vi "Get Features DB.vi"(6 "Local Data in":T3, 7 "UI References":T1, 8 "error in (no error)":errorcluster, 10 "Action":T2=enum."Get Preview", 11 "Mouse Position (Start)":cluster{"X":i32, "Y":i32}) -> (0 "error out":errorcluster, 1 "Refresh?":bool, 2 "Features":string[][](array[string]), 3 "FTR Names":string[](array[string]), 4 "Local Data out":T3)   [LabVIEW 2024]
uses:
  Controls/RVHR - Local Data.ctl
  Controls/Test Cluster.ctl
  Controls/Excluded Information.ctl
  Controls/Language.ctl
  Controls/Device_Type.ctl
  <vilib>/Utility/miscctls.llb/LVRectTypeDef.ctl
  <vilib>/Utility/miscctls.llb/LVBoundsTypeDef.ctl
  Controls/DB Manager Commands.ctl
  Controls/RVHR - UI Refs.ctl
  Controls/Run Listbox Command.ctl
  <vilib>/drjdpowell/SQLite Library/SQL Connection/Open (path).vi
  <vilib>/drjdpowell/SQLite Library/SQL Connection/Open (string).vi
  <vilib>/AdvancedString/Path To Command Line String.vi
  <vilib>/drjdpowell/SQLite Library/SQL Connection/Execute SQL (Single Integer).vi
  <vilib>/drjdpowell/SQLite Library/SQL Connection/Execute SQL.vi
  <vilib>/drjdpowell/SQLite Library/SQL Connection/Execute SQL (1D String).vi
  <vilib>/drjdpowell/SQLite Library/SQL Connection/Execute SQL (No results).vi
  <vilib>/drjdpowell/SQLite Library/SQL Connection/Connection.lvclass
  <vilib>/drjdpowell/SQLite Library/SQLite.lvlib
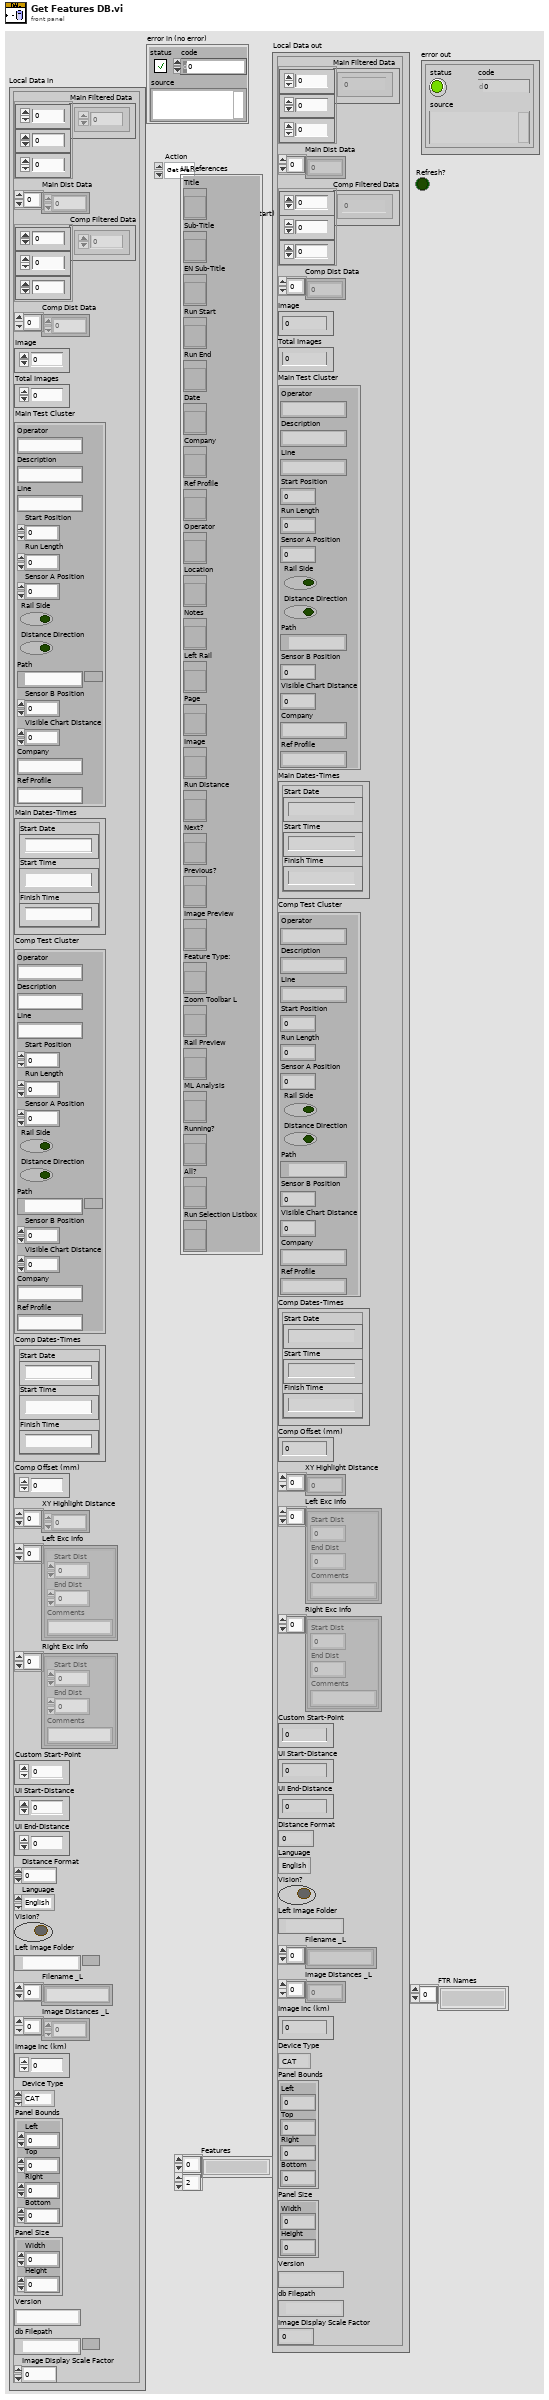
[diagram p1: front panel]
types:
  T1 = typedef "RVHR - UI Refs.ctl" = cluster{"Title":refnum<vi>, "Sub-Title":refnum<vi>, "EN Sub-Title":refnum<vi>, "Run Start":refnum<vi>, "Run End":refnum<vi>, "Date":refnum<vi>, "Company":refnum<vi>, "Ref Profile":refnum<vi>, "Operator":refnum<vi>, "Location":refnum<vi>, "Notes":refnum<vi>, "Left Rail":refnum<vi>, "Page":refnum<vi>, "Image":refnum<vi>, "Run Distance":refnum<vi>, "Next?":refnum<vi>, "Previous?":refnum<vi>, "Image Preview":refnum<vi>, "Feature Type:":refnum<vi>, "Zoom Toolbar L":refnum<vi>, "Rail Preview":refnum<vi>, "ML Analysis":refnum<vi>, "Running?":refnum<vi>, "All?":refnum<vi>, "Run Selection Listbox":refnum<vi>}
  T2 = typedef "DB Manager Commands.ctl" = enum16{"Get Image", "Get Preview", "Add", "Remove", "Update", "Get FTR Names"}
  T3 = typedef "RVHR - Local Data.ctl" = cluster{"Main Filtered Data":dbl[][][], "Main Dist Data":dbl[], "Comp Filtered Data":dbl[][][], "Comp Dist Data":dbl[], "Image":u16, "Total Images":u16, "Main Test Cluster":T4, "Main Dates-Times":cluster{"Start Date":string, "Start Time":string, "Finish Time":string}, "Comp Test Cluster":T4, "Comp Dates-Times":cluster{"Start Date":string, "Start Time":string, "Finish Time":string}, "Comp Offset (mm)":i64, "XY Highlight Distance":dbl[], "Left Exc Info":T5[], "Right Exc Info":T5[], "Custom Start-Point":dbl, "UI Start-Distance":dbl, "UI End-Distance":dbl, "Distance Format":u8, "Language":T6, "Vision?":bool, "Left Image Folder":path, "Filename _L":string[], "Image Distances _L":dbl[], "Image Inc (km)":dbl, "Device Type":T7, "Panel Bounds":T8, "Panel Size":T9, "Version":string, "db Filepath":path, "Image Display Scale Factor":dbl}
  T4 = typedef "Test Cluster.ctl" = cluster{"Operator":string, "Description":string, "Line":string, "Start Position":dbl, "Run Length":dbl, "Sensor A Position":dbl, "Rail Side":bool, "Distance Direction":bool, "Path":path, "Sensor B Position":dbl, "Visible Chart Distance":dbl, "Company":string, "Ref Profile":string}
  T5 = typedef "Excluded Information.ctl" = cluster{"Start Dist":dbl, "End Dist":dbl, "Comments":string}
  T6 = typedef "Language.ctl" = enum16{"English", "Chinese", "German"}
  T7 = typedef "Device_Type.ctl" = enum16{"CAT", "Bi-CAT", "YRCA", "RCA", "RV-HR", "TV-HR"}
  T8 = typedef "LVRectTypeDef.ctl" = cluster{"Left":i16, "Top":i16, "Right":i16, "Bottom":i16}
  T9 = typedef "LVBoundsTypeDef.ctl" = cluster{"Width":u32, "Height":u32}
  T10 = typedef "Run Listbox Command.ctl" = enum16{"Init", "Item Names", "Update", "Update All", "Get Selections", "Clear"}
  T11 = typedef "LVMouseTypeDef.ctl" = cluster{"Mouse Position":cluster{"X":i32, "Y":i32}, "Mouse Modifiers":cluster{"Button Down":bool, "Shift Mod":bool, "Menu Mod":bool, "Option Mod":bool}}
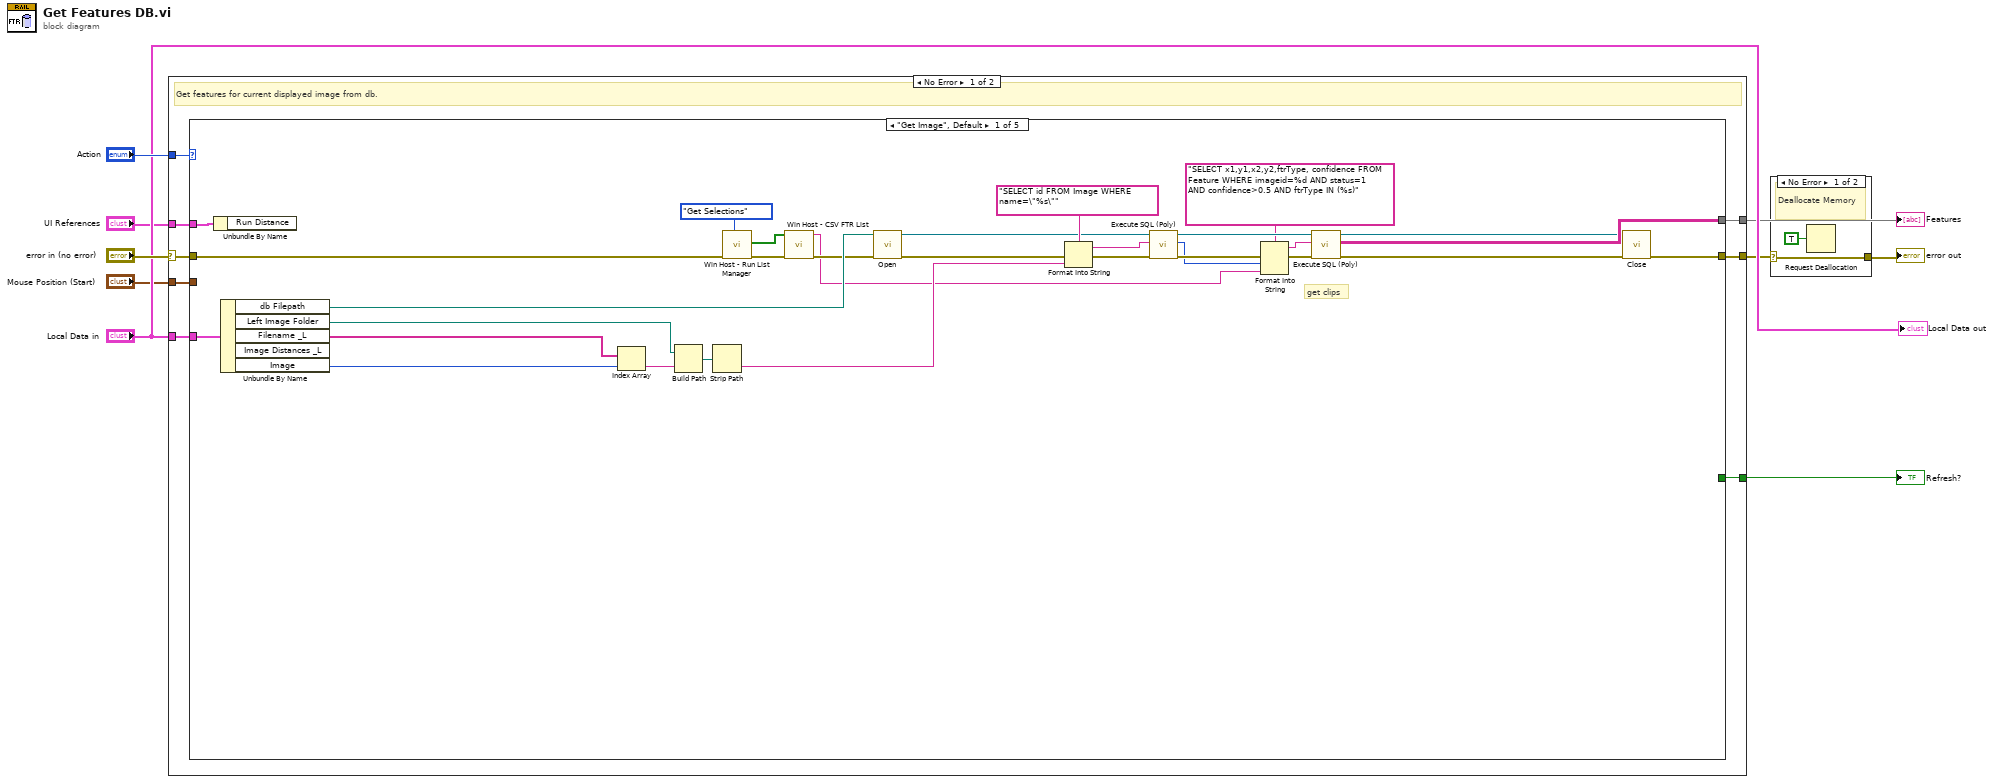
[diagram p0: block diagram]
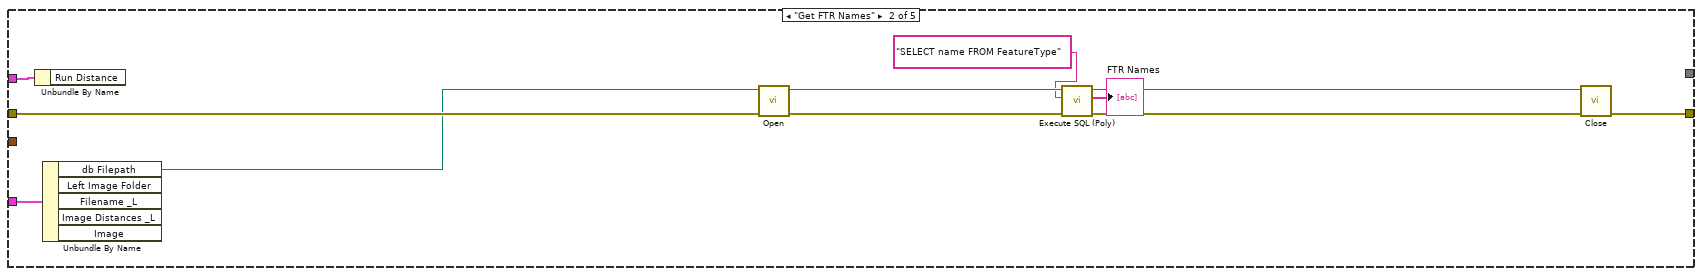
[diagram p3: hidden frame]
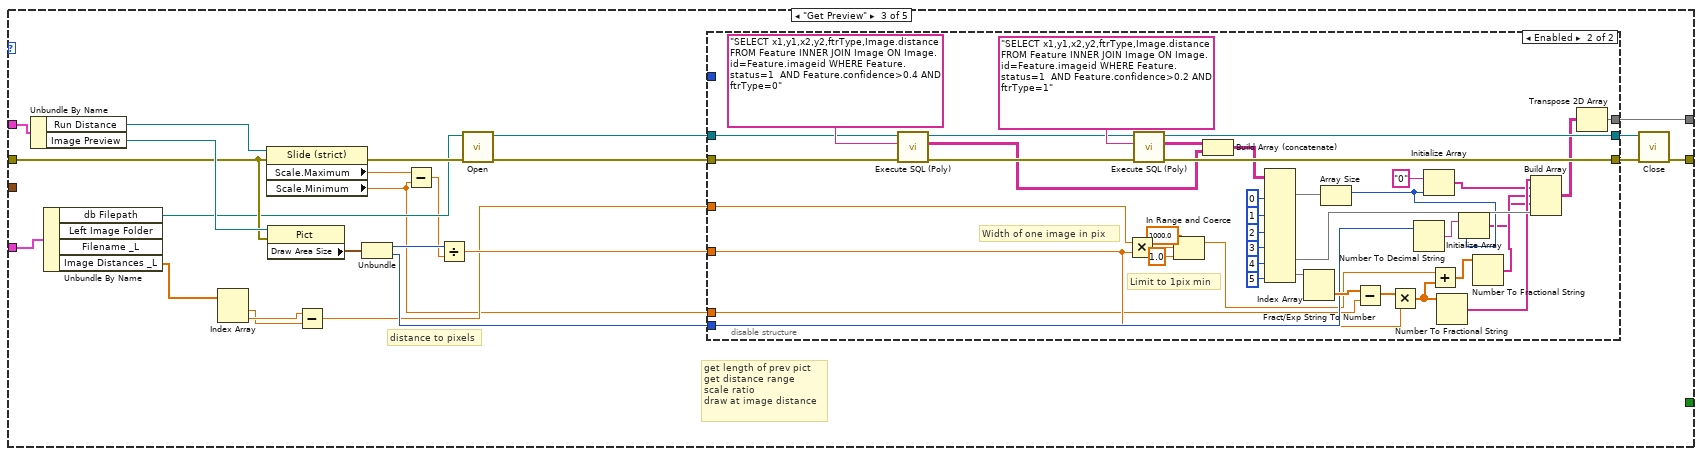
[diagram p4: hidden frame]
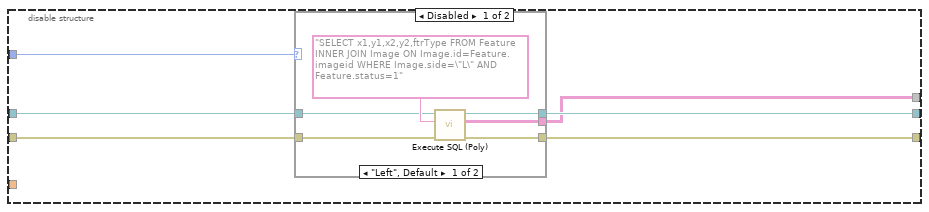
[diagram p5: hidden frame]
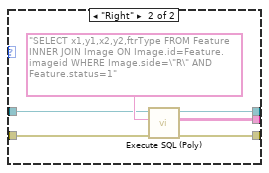
[diagram p6: hidden frame]
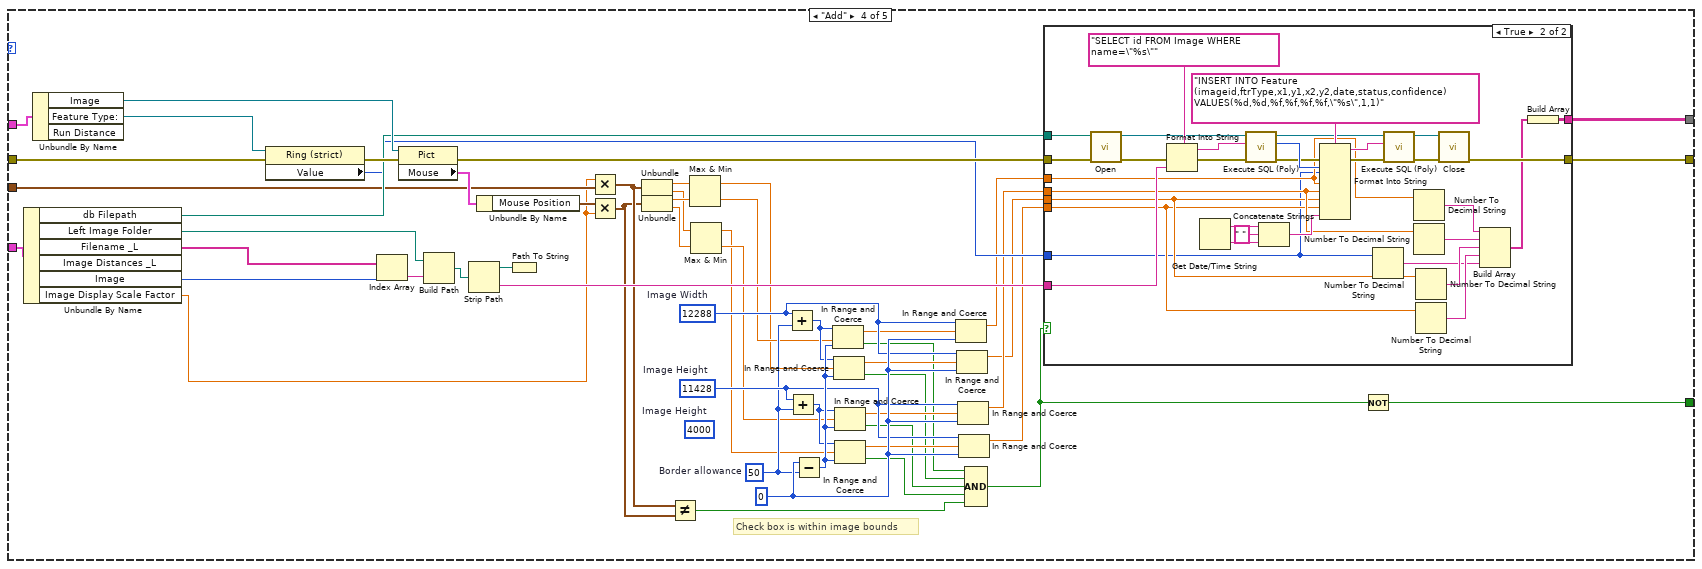
[diagram p7: hidden frame]
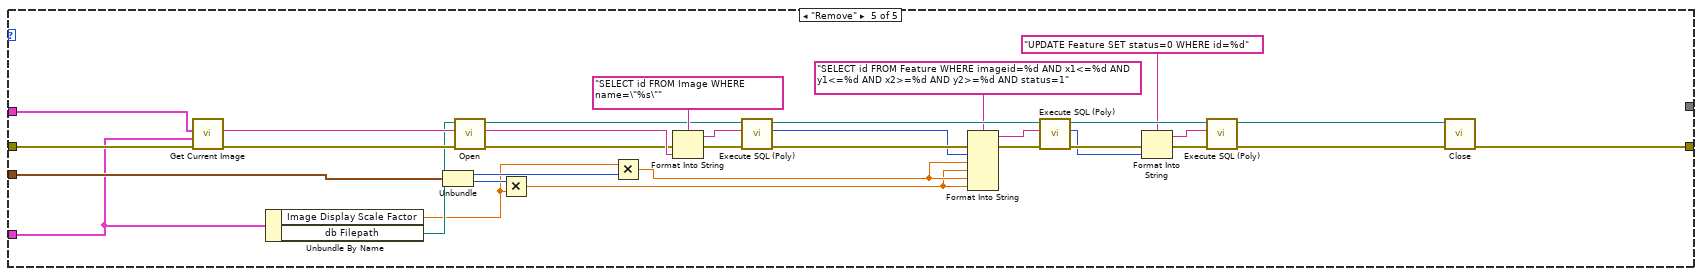
[diagram p9: hidden frame]
diagram:
  n1 = case shown="No Error" "error in (no error)" {
    selector: "error in (no error)" -> [w17 w262]
    tunnel: "Local Data in" -> [w15 _]
    tunnel: [w16 w262] -> w2
    tunnel: "Action" -> [w14 _]
    tunnel: "Mouse Position (Start)" -> [w13 _]
    tunnel: "UI References" -> [w12 _]
    tunnel: [w11 _] -> w4
    tunnel: [w10 _] -> w3
    frame No Error {
      # "Get features for current displayed image from db."
      n2 = case shown="\"Get Image\", Default" w14 {
        tunnel: w17 -> [w21 w51 w71 w180 w238]
        tunnel: [w47 w58 w82 w195 w261] -> w16
        tunnel: w15 -> [w46 w57 w81 w194 w236]
        tunnel: w13 -> [_ _ _ w172 w260]
        tunnel: w12 -> [w31 w52 w75 w190 w239]
        tunnel: [w27 _ w76 w181 _] -> w11
        tunnel: [_ _ _ w173 _] -> w10
        frame "Get Image", Default {
          # "get clips"
          n3 = Unbundle By Name(w31) -> ()  [unwired: 1 out]
          n4 = Unbundle By Name(w46) -> ("db Filepath"=w30:path, "Left Image Folder"=w45:path, "Filename _L"=w44:string[], "Image"=w24:u16)  [unwired: 1 out]
          n5 = Index Array(array=w44, index=w24) -> (element=w43:string)
          n6 = Build Path(base path=w45, name or relative path=w43) -> (appended path=w42:path)
          n7 = Strip Path(path=w42) -> (name=w38:string)  [unwired: 1 out]
          n8 = call "Win Host - Run List Manager.vi"("Command"=Run_Listbox_Command."Get Selections", "error in (no error)"=w21) -> ("error out"=w20:errorcluster, "Selected Runs?"=w22:bool[])  [unwired: 6 in, 2 out]
          n9 = call "Win Host - CSV FTR List.vi"("error in (no error)"=w20, "Selected Runs?"=w22) -> ("error out"=w19:errorcluster, "ftrTypes csv"=w18:string)  [unwired: 8 in]
          n10 = call-poly <vilib>:"Open.vi"("error in (no error)"=w19, "db file"=w30) -> ("error out"=w35:errorcluster, "SQLite Connection"=w39:refnum<class "Connection.lvclass">)  [unwired: 8 in]
          n11 = Format Into String(format string="SELECT id FROM Image WHERE name=\"%s\"", error in=w35, w38) -> (resulting string=w40:string, error out=w37:errorcluster)  [unwired: 1 in]
          n12 = call-poly <vilib>:"Execute SQL (Poly).vi"("error in (no error)"=w37, "SQL"=w40, "SQLite Connection in"=w39) -> ("error out"=w36:errorcluster, "Result"=w26:i64, "SQLite Connection"=w34:refnum<class "Connection.lvclass">)  [unwired: 6 in]
          n13 = Format Into String(format string="SELECT x1,y1,x2,y2,ftrType, confidence FROM Feature WHERE imageid=%d AND status=1 AND confidence>0.5 AND ftrType IN (%s)", error in=w36, w26, w18) -> (resulting string=w32:string, error out=w33:errorcluster)  [unwired: 1 in]
          n14 = call-poly <vilib>:"Execute SQL (Poly).vi"("error in (no error)"=w33, "SQL"=w32, "SQLite Connection in"=w34) -> ("error out"=w29:errorcluster, "Result Set"=w27:string[][], "SQLite Connection"=w25:refnum<class "Connection.lvclass">)  [unwired: 5 in, 1 out]
          n15 = call-dynamic "Close.vi"("error in (no error)"=w29, "SQLite Connection in"=w25) -> ("error out"=w47:errorcluster)  [unwired: 9 in]
        }
        frame "Get FTR Names" {
          n16 = Unbundle By Name(w52) -> ()  [unwired: 1 out]
          n17 = Unbundle By Name(w57) -> ("db Filepath"=w50:path)  [unwired: 4 out]
          n18 = call-poly <vilib>:"Open.vi"("error in (no error)"=w51, "db file"=w50) -> ("error out"=w54:errorcluster, "SQLite Connection"=w56:refnum<class "Connection.lvclass">)  [unwired: 8 in]
          n19 = call-poly <vilib>:"Execute SQL (Poly).vi"("error in (no error)"=w54, "SQL"="SELECT name FROM FeatureType" ("format string"), "SQLite Connection in"=w56) -> ("error out"=w55:errorcluster, "Result Set"=→"FTR Names":string[], "SQLite Connection"=w53:refnum<class "Connection.lvclass">)  [unwired: 5 in, 1 out]
          n20 = call-dynamic "Close.vi"("error in (no error)"=w55, "SQLite Connection in"=w53) -> ("error out"=w58:errorcluster)  [unwired: 9 in]
        }
        frame "Get Preview" {
          # "get length of prev pict\nget distance range\nscale ratio\ndraw at image distance"
          # "distance to pixels"
          n21 = Unbundle By Name(w75) -> ("Run Distance"=w74:refnum<vi>, "Image Preview"=w72:refnum<vi>)
          n22 = Unbundle By Name(w81) -> ("db Filepath"=w62:path, "Image Distances _L"=w66:dbl[])  [unwired: 2 out]
          n23 = Index Array(array=w66) -> (element #1=w64:dbl, element #2=w65:dbl)  [unwired: 2 in]
          n24 = property class="Slide (strict)"(reference=w74, error in=w71) -> (error out=w73:errorcluster, "Scale.Maximum"=w61:dbl, "Scale.Minimum"=w59:dbl)  [unwired: 1 out]
          n25 = property class="Pict"(reference=w72, error in=w71) -> ("Draw Area Size"=w70:T9)  [unwired: 2 out]
          n26 = Subtract(x=w65, y=w64) -> (x-y=w63:dbl)
          n27 = Unbundle(w70) -> ("Width"=w69:u32, "Height"=w67:u32)
          n28 = Subtract(x=w61, y=w59) -> (x-y=w60:dbl)
          n29 = Divide(x=w69, y=w60) -> (x/y=w68:dbl)
          n30 = call-poly <vilib>:"Open.vi"("error in (no error)"=w73, "db file"=w62) -> ("error out"=w80:errorcluster, "SQLite Connection"=w79:refnum<class "Connection.lvclass">)  [unwired: 8 in]
          n31 = disable-structure shown="Enabled" {
            disable-tunnel: w80 -> [w88 w106]
            disable-tunnel: w79 -> [w87 w107]
            disable-tunnel: [w86 w141] -> w78
            disable-tunnel: [w85 w140] -> w77
            disable-tunnel: [w84 w119] -> w76
            disable-tunnel: _ -> [w83 _]
            disable-tunnel: w68 -> [_ w116]
            disable-tunnel: w67 -> [_ w136]
            disable-tunnel: w63 -> [_ w117]
            disable-tunnel: w59 -> [_ w114]
            frame Disabled {
              n32 = case shown="\"Left\", Default" w83 {
                tunnel: w88 -> [w93 w99]
                tunnel: w87 -> [w92 w98]
                tunnel: [w91 w97] -> w86
                tunnel: [w90 w96] -> w85
                tunnel: [w89 w95] -> w84
                frame "Left", Default {
                  n33 = call-poly <vilib>:"Execute SQL (Poly).vi"("error in (no error)"=w93, "SQL"="SELECT x1,y1,x2,y2,ftrType FROM Feature INNER JOIN Image ON Image.id=Feature.imageid WHERE Image.side=\"L\" AND Feature.status=1" ("format string"), "SQLite Connection in"=w92) -> ("error out"=w90:errorcluster, "Result Set"=w89:string[][], "SQLite Connection"=w91:refnum<class "Connection.lvclass">)  [unwired: 5 in, 1 out]
                }
                frame "Right" {
                  n34 = call-poly <vilib>:"Execute SQL (Poly).vi"("error in (no error)"=w99, "SQL"="SELECT x1,y1,x2,y2,ftrType FROM Feature INNER JOIN Image ON Image.id=Feature.imageid WHERE Image.side=\"R\" AND Feature.status=1" ("format string"), "SQLite Connection in"=w98) -> ("error out"=w96:errorcluster, "Result Set"=w95:string[][], "SQLite Connection"=w97:refnum<class "Connection.lvclass">)  [unwired: 5 in, 1 out]
                }
              }
            }
            frame Enabled {
              # "Limit to 1pix min"
              # "Width of one image in pix"
              n35 = call-poly <vilib>:"Execute SQL (Poly).vi"("error in (no error)"=w106, "SQL"="SELECT x1,y1,x2,y2,ftrType,Image.distance FROM Feature INNER JOIN Image ON Image.id=Feature.imageid WHERE Feature.status=1  AND Feature.confidence>0.4 AND ftrType=0" ("format string"), "SQLite Connection in"=w107) -> ("error out"=w105:errorcluster, "Result Set"=w102:string[][], "SQLite Connection"=w104:refnum<class "Connection.lvclass">)  [unwired: 5 in, 1 out]
              n36 = Multiply(x=w117, y=w116) -> (x*y=w113:dbl)
              n37 = call-poly <vilib>:"Execute SQL (Poly).vi"("error in (no error)"=w105, "SQL"="SELECT x1,y1,x2,y2,ftrType,Image.distance FROM Feature INNER JOIN Image ON Image.id=Feature.imageid WHERE Feature.status=1  AND Feature.confidence>0.2 AND ftrType=1" ("format string"), "SQLite Connection in"=w104) -> ("error out"=w140:errorcluster, "Result Set"=w103:string[][], "SQLite Connection"=w141:refnum<class "Connection.lvclass">)  [unwired: 5 in, 1 out]
              n38 = In Range and Coerce(upper limit=1000.0, x=w113, lower limit=1.0) -> (coerced(x)=w111:dbl)  [unwired: 1 out]
              n39 = Build Array (concatenate)(w103, w102) -> (w101:string[][])
              n40 = Index Array(array=w101, index (col) #1=0 ("disabled index (col)"), index (col) #2=1 ("index (col)"), index (col) #3=2 ("index (col)"), index (col) #4=3 ("index (col)"), index (col) #5=4 ("index (col)"), index (col) #6=5 ("index (col)")) -> (element #1=w131:string[], element #5=w134:string[], element #6=w139:string[])  [unwired: 6 in, 3 out]
              n41 = Fract/Exp String To Number(string=w139) -> (number=w138:dbl[])  [unwired: 3 in, 1 out]
              n42 = Array Size(array=w131) -> (size(s)=w127:i32)
              n43 = Subtract(x=w138, y=w114) -> (x-y=w115:dbl[])
              n44 = Multiply(x=w115, y=w116) -> (x*y=w137:dbl[])
              n45 = Number To Decimal String(number=w136) -> (decimal integer string=w128:string)  [unwired: 1 in]
              n46 = Initialize Array("0" ("string"), w127) -> (w129:string[])
              n47 = Add(x=w111, y=w137) -> (x+y=w135:dbl[])
              n48 = Number To Fractional String(number=w137) -> (F-format string=w133:string[])  [unwired: 3 in]
              n49 = Initialize Array(w128, w127) -> (w126:string[])
              n50 = Number To Fractional String(number=w135) -> (F-format string=w132:string[])  [unwired: 3 in]
              n51 = Build Array(w133, w129, w132, w126, w134) -> (w118:string[][])
              n52 = Transpose 2D Array(2D array=w118) -> (transposed array=w119:string[][])
            }
          }
          n53 = call-dynamic "Close.vi"("error in (no error)"=w77, "SQLite Connection in"=w78) -> ("error out"=w82:errorcluster)  [unwired: 9 in]
        }
        frame "Add" {
          (unwired) 4000  # Image Height
          w157 = 50  # Border allowance
          w165 = 11428  # Image Height
          w164 = 12288  # Image Width
          w167 = 0 ("y")
          # "Check box is within image bounds"
          n54 = Unbundle By Name(w194) -> ("db Filepath"=w175:path, "Left Image Folder"=w193:path, "Filename _L"=w192:string[], "Image"=w142:u16, "Image Display Scale Factor"=w168:dbl)  [unwired: 1 out]
          n55 = Unbundle By Name(w190) -> ("Image"=w189:refnum<vi>, "Feature Type:"=w183:refnum<vi>)  [unwired: 1 out]
          n56 = property class="Ring (strict)"(reference=w183, error in=w180) -> (error out=w182:errorcluster, "Value"=w174:u16)  [unwired: 1 out]
          n57 = Index Array(array=w192, index=w142) -> (element=w191:string)
          n58 = property class="Pict"(reference=w189, error in=w182) -> (error out=w184:errorcluster, "Mouse"=w185:T11)  [unwired: 1 out]
          n59 = Build Path(base path=w193, name or relative path=w191) -> (appended path=w188:path)
          n60 = Strip Path(path=w188) -> (stripped path=w187:path, name=w186:string)
          n61 = Unbundle By Name(w185) -> ("Mouse Position"=w170:cluster{"X":i32, "Y":i32})
          n62 = Path To String(path=w187) -> ()  [unwired: 1 out]
          n63 = Multiply(x=w168, y=w172) -> (x*y=w171:cluster{"X":dbl, "Y":dbl})
          n64 = Multiply(x=w170, y=w168) -> (x*y=w169:cluster{"X":dbl, "Y":dbl})
          n65 = Unbundle(w171) -> ("X"=w179:dbl, "Y"=w177:dbl)
          n66 = Unbundle(w169) -> ("X"=w178:dbl, "Y"=w176:dbl)
          n67 = Not Equal?(x=w171, y=w169) -> (x != y?=w152:bool)
          n68 = Max & Min(x=w179, y=w178) -> (max(x,y)=w146:dbl, min(x,y)=w151:dbl)
          n69 = Max & Min(x=w177, y=w176) -> (max(x,y)=w148:dbl, min(x,y)=w149:dbl)
          n70 = Add(x=w164, y=w157) -> (x+y=w162:i32)
          n71 = Add(x=w165, y=w157) -> (x+y=w163:i32)
          n72 = Subtract(x=w167, y=w157) -> (x-y=w166:i32)
          n73 = In Range and Coerce(upper limit=w162, x=w151, lower limit=w166) -> (coerced(x)=w161:dbl, In Range?=w156:bool)
          n74 = In Range and Coerce(upper limit=w162, x=w146, lower limit=w166) -> (coerced(x)=w160:dbl, In Range?=w155:bool)
          n75 = In Range and Coerce(upper limit=w163, x=w149, lower limit=w166) -> (coerced(x)=w159:dbl, In Range?=w154:bool)
          n76 = In Range and Coerce(upper limit=w163, x=w148, lower limit=w166) -> (coerced(x)=w158:dbl, In Range?=w153:bool)
          n77 = In Range and Coerce(upper limit=w164, x=w161, lower limit=w167) -> (coerced(x)=w150:dbl)  [unwired: 1 out]
          n78 = In Range and Coerce(upper limit=w164, x=w160, lower limit=w167) -> (coerced(x)=w145:dbl)  [unwired: 1 out]
          n79 = In Range and Coerce(upper limit=w165, x=w159, lower limit=w167) -> (coerced(x)=w147:dbl)  [unwired: 1 out]
          n80 = In Range and Coerce(upper limit=w165, x=w158, lower limit=w167) -> (coerced(x)=w144:dbl)  [unwired: 1 out]
          n81 = Compound Arithmetic op=AND(w156, w155, w154, w153, w152) -> (w143:bool)
          n82 = case shown="True" w143 {
            tunnel: [w196 w226] -> w195
            tunnel: w175 -> [_ w225]
            tunnel: w186 -> [_ w213]
            tunnel: w184 -> [w196 w209]
            tunnel: [_ w203] -> w181
            tunnel: w150 -> [_ w202]
            tunnel: w147 -> [_ w201]
            tunnel: w145 -> [_ w200]
            tunnel: w144 -> [_ w199]
            tunnel: w174 -> [_ w197]
            frame False {
            }
            frame True {
              n83 = call-poly <vilib>:"Open.vi"("error in (no error)"=w209, "db file"=w225) -> ("error out"=w210:errorcluster, "SQLite Connection"=w216:refnum<class "Connection.lvclass">)  [unwired: 8 in]
              n84 = Format Into String(format string="SELECT id FROM Image WHERE name=\"%s\"", error in=w210, w213) -> (resulting string=w217:string, error out=w212:errorcluster)  [unwired: 1 in]
              n85 = Get Date/Time String() -> (date string=w222:string, time string=w221:string)  [unwired: 3 in]
              n86 = call-poly <vilib>:"Execute SQL (Poly).vi"("error in (no error)"=w212, "SQL"=w217, "SQLite Connection in"=w216) -> ("error out"=w211:errorcluster, "Result"=w214:i64, "SQLite Connection"=w215:refnum<class "Connection.lvclass">)  [unwired: 6 in]
              n87 = Concatenate Strings(w222, " " ("string"), w221) -> (w219:string)
              n88 = Format Into String(format string="INSERT INTO Feature (imageid,ftrType,x1,y1,x2,y2,date,status,confidence) VALUES(%d,%d,%f,%f,%f,%f,\"%s\",1,1)", error in=w211, w214, w197, w202, w201, w200, w199, w219) -> (resulting string=w224:string, error out=w228:errorcluster)  [unwired: 1 in]
              n89 = Number To Decimal String(number=w197) -> (decimal integer string=w198:string)  [unwired: 1 in]
              n90 = call-poly <vilib>:"Execute SQL (Poly).vi"("error in (no error)"=w228, "SQL"=w224, "SQLite Connection in"=w215) -> ("error out"=w229:errorcluster, "SQLite Connection"=w227:refnum<class "Connection.lvclass">)  [unwired: 7 in]
              n91 = Number To Decimal String(number=w202) -> (decimal integer string=w204:string)  [unwired: 1 in]
              n92 = Number To Decimal String(number=w201) -> (decimal integer string=w205:string)  [unwired: 1 in]
              n93 = Number To Decimal String(number=w200) -> (decimal integer string=w206:string)  [unwired: 1 in]
              n94 = Number To Decimal String(number=w199) -> (decimal integer string=w207:string)  [unwired: 1 in]
              n95 = call-dynamic "Close.vi"("error in (no error)"=w229, "SQLite Connection in"=w227) -> ("error out"=w226:errorcluster)  [unwired: 9 in]
              n96 = Build Array(w204, w205, w206, w207, w198) -> (w208:string[])
              n97 = Build Array(w208) -> (w203:string[][])
            }
          }
          n98 = Not(x=w143) -> (.not. x?=w173:bool)
        }
        frame "Remove" {
          n99 = call "Get Current Image.vi"("error in (no error)"=w238, "Local Data in"=w236, "UI References"=w239) -> ("error out"=w237:errorcluster, "Current Image"=w253:string)  [unwired: 7 in]
          n100 = Unbundle By Name(w236) -> ("Image Display Scale Factor"=w230:dbl, "db Filepath"=w235:path)
          n101 = Unbundle(w260) -> ("X"=w233:i32, "Y"=w234:i32)
          n102 = call-poly <vilib>:"Open.vi"("error in (no error)"=w237, "db file"=w235) -> ("error out"=w250:errorcluster, "SQLite Connection"=w255:refnum<class "Connection.lvclass">)  [unwired: 8 in]
          n103 = Multiply(x=w234, y=w230) -> (x*y=w231:dbl)
          n104 = Multiply(x=w230, y=w233) -> (x*y=w232:dbl)
          n105 = Format Into String(format string="SELECT id FROM Image WHERE name=\"%s\"", error in=w250, w253) -> (resulting string=w256:string, error out=w252:errorcluster)  [unwired: 1 in]
          n106 = call-poly <vilib>:"Execute SQL (Poly).vi"("error in (no error)"=w252, "SQL"=w256, "SQLite Connection in"=w255) -> ("error out"=w251:errorcluster, "Result"=w243:i64, "SQLite Connection"=w254:refnum<class "Connection.lvclass">)  [unwired: 6 in]
          n107 = Format Into String(format string="SELECT id FROM Feature WHERE imageid=%d AND x1<=%d AND y1<=%d AND x2>=%d AND y2>=%d AND status=1", error in=w251, w243, w232, w231, w232, w231) -> (resulting string=w258:string, error out=w259:errorcluster)  [unwired: 1 in]
          n108 = call-poly <vilib>:"Execute SQL (Poly).vi"("error in (no error)"=w259, "SQL"=w258, "SQLite Connection in"=w254) -> ("error out"=w246:errorcluster, "Result"=w240:i64, "SQLite Connection"=w248:refnum<class "Connection.lvclass">)  [unwired: 6 in]
          n109 = Format Into String(format string="UPDATE Feature SET status=0 WHERE id=%d", error in=w246, w240) -> (resulting string=w241:string, error out=w245:errorcluster)  [unwired: 1 in]
          n110 = call-poly <vilib>:"Execute SQL (Poly).vi"("error in (no error)"=w245, "SQL"=w241, "SQLite Connection in"=w248) -> ("error out"=w244:errorcluster, "SQLite Connection"=w247:refnum<class "Connection.lvclass">)  [unwired: 7 in]
          n111 = call-dynamic "Close.vi"("error in (no error)"=w244, "SQLite Connection in"=w247) -> ("error out"=w261:errorcluster)  [unwired: 9 in]
        }
      }
    }
    frame Error {
    }
  }
  "Features" <- w4
  "Refresh?" <- w3
  n112 = case shown="No Error" w2 {
    selector: w2 -> [w263 w265]
    tunnel: [w263 w265] -> w1
    frame No Error {
      # "Deallocate Memory"
      n113 = Request Deallocation(TRUE ("flag")) -> ()
    }
    frame Error {
    }
  }
  "error out" <- w1
  "Local Data out" <- "Local Data in"
